vi "App - analyze RUS V6.vi"() -> ()   [LabVIEW 2015] (continued)
CO22__130814c/5_Cooling_2nd_try/September_2014/091614/117.62100K_500_2500_2.10000V_0.00000T_Sep16-2014__20-07-41_001_091614.bin", "last mod"=timestamp(3493757261 s since 1904-01-01), "file name str"="D:\\Data\\Ultrasound\\LSCO\\LSCO22__130814c\\5_Cooling_2nd_try\\September_2014\\091614\\117.62100K_500_2500_2.10000V_0.00000T_Sep16-2014__20-07-41_001_091614.bin", "mod time(min)"=58229287.68333333, "file format"=enum."binary", "power(V)"=2.1, "Magn Field(T) "=0.0}, {"temperature"=117.382, "temperature str"="117.38200", "file path"=path "D:/Data/Ultrasound/LSCO/LSCO22__130814c/5_Cooling_2nd_try/September_2014/091614/117.38200K_500_2500_2.10000V_0.00000T_Sep16-2014__20-09-01_001_091614.bin", "last mod"=timestamp(3493757341 s since 1904-01-01), "file name str"="D:\\Data\\Ultrasound\\LSCO\\LSCO22__130814c\\5_Cooling_2nd_try\\September_2014\\091614\\117.38200K_500_2500_2.10000V_0.00000T_Sep16-2014__20-09-01_001_091614.bin", "mod time(min)"=58229289.016666666, "file format"=enum."binary", "power(V)"=2.1, "Magn Field(T) "=0.0}, {"temperature"=117.138, "temperature str"="117.13800", "file path"=path "D:/Data/Ultrasound/LSCO/LSCO22__130814c/5_Cooling_2nd_try/September_2014/091614/117.13800K_500_2500_2.10000V_0.00000T_Sep16-2014__20-10-20_001_091614.bin", "last mod"=timestamp(3493757420 s since 1904-01-01), "file name str"="D:\\Data\\Ultrasound\\LSCO\\LSCO22__130814c\\5_Cooling_2nd_try\\September_2014\\091614\\117.13800K_500_2500_2.10000V_0.00000T_Sep16-2014__20-10-20_001_091614.bin", "mod time(min)"=58229290.333333336, "file format"=enum."binary", "power(V)"=2.1, "Magn Field(T) "=0.0}, {"temperature"=116.892, "temperature str"="116.89200", "file path"=path "D:/Data/Ultrasound/LSCO/LSCO22__130814c/5_Cooling_2nd_try/September_2014/091614/116.89200K_500_2500_2.10000V_0.00000T_Sep16-2014__20-11-40_001_091614.bin", "last mod"=timestamp(3493757500 s since 1904-01-01), "file name str"="D:\\Data\\Ultrasound\\LSCO\\LSCO22__130814c\\5_Cooling_2nd_try\\September_2014\\091614\\116.89200K_500_2500_2.10000V_0.00000T_Sep16-2014__20-11-40_001_091614.bin", "mod time(min)"=58229291.666666664, "file format"=enum."binary", "power(V)"=2.1, "Magn Field(T) "=0.0}, {"temperature"=116.657, "temperature str"="116.65700", "file path"=path "D:/Data/Ultrasound/LSCO/LSCO22__130814c/5_Cooling_2nd_try/September_2014/091614/116.65700K_500_2500_2.10000V_0.00000T_Sep16-2014__20-12-59_001_091614.bin", "last mod"=timestamp(3493757579 s since 1904-01-01), "file name str"="D:\\Data\\Ultrasound\\LSCO\\LSCO22__130814c\\5_Cooling_2nd_try\\September_2014\\091614\\116.65700K_500_2500_2.10000V_0.00000T_Sep16-2014__20-12-59_001_091614.bin", "mod time(min)"=58229292.983333334, "file format"=enum."binary", "power(V)"=2.1, "Magn Field(T) "=0.0}, {"temperature"=116.414, "temperature str"="116.41400", "file path"=path "D:/Data/Ultrasound/LSCO/LSCO22__130814c/5_Cooling_2nd_try/September_2014/091614/116.41400K_500_2500_2.10000V_0.00000T_Sep16-2014__20-14-18_001_091614.bin", "last mod"=timestamp(3493757658 s since 1904-01-01), "file name str"="D:\\Data\\Ultrasound\\LSCO\\LSCO22__130814c\\5_Cooling_2nd_try\\September_2014\\091614\\116.41400K_500_2500_2.10000V_0.00000T_Sep16-2014__20-14-18_001_091614.bin", "mod time(min)"=58229294.3, "file format"=enum."binary", "power(V)"=2.1, "Magn Field(T) "=0.0}, {"temperature"=116.182, "temperature str"="116.18200", "file path"=path "D:/Data/Ultrasound/LSCO/LSCO22__130814c/5_Cooling_2nd_try/September_2014/091614/116.18200K_500_2500_2.10000V_0.00000T_Sep16-2014__20-15-38_001_091614.bin", "last mod"=timestamp(3493757738 s since 1904-01-01), "file name str"="D:\\Data\\Ultrasound\\LSCO\\LSCO22__130814c\\5_Cooling_2nd_try\\September_2014\\091614\\116.18200K_500_2500_2.10000V_0.00000T_Sep16-2014__20-15-38_001_091614.bin", "mod time(min)"=58229295.63333333, "file format"=enum."binary", "power(V)"=2.1, "Magn Field(T) "=0.0}, {"temperature"=115.94, "temperature str"="115.94000", "file path"=path "D:/Data/Ultrasound/LSCO/LSCO22__130814c/5_Cooling_2nd_try/September_2014/091614/115.94000K_500_2500_2.10000V_0.00000T_Sep16-2014__20-16-57_001_091614.bin", "last mod"=timestamp(3493757817 s since 1904-01-01), "file name str"="D:\\Data\\Ultrasound\\LSCO\\LSCO22__130814c\\5_Cooling_2nd_try\\September_2014\\091614\\115.94000K_500_2500_2.10000V_0.00000T_Sep16-2014__20-16-57_001_091614.bin", "mod time(min)"=58229296.95, "file format"=enum."binary", "power(V)"=2.1, "Magn Field(T) "=0.0}, {"temperature"=115.7, "temperature str"="115.70000", "file path"=path "D:/Data/Ultrasound/LSCO/LSCO22__130814c/5_Cooling_2nd_try/September_2014/091614/115.70000K_500_2500_2.10000V_0.00000T_Sep16-2014__20-18-16_001_091614.bin", "last mod"=timestamp(3493757896 s since 1904-01-01), "file name str"="D:\\Data\\Ultrasound\\LSCO\\LSCO22__130814c\\5_Cooling_2nd_try\\September_2014\\091614\\115.70000K_500_2500_2.10000V_0.00000T_Sep16-2014__20-18-16_001_091614.bin", "mod time(min)"=58229298.266666666, "file format"=enum."binary", "power(V)"=2.1, "Magn Field(T) "=0.0}, {"temperature"=115.472, "temperature str"="115.47200", "file path"=path "D:/Data/Ultrasound/LSCO/LSCO22__130814c/5_Cooling_2nd_try/September_2014/091614/115.47200K_500_2500_2.10000V_0.00000T_Sep16-2014__20-19-36_001_091614.bin", "last mod"=timestamp(3493757976 s since 1904-01-01), "file name str"="D:\\Data\\Ultrasound\\LSCO\\LSCO22__130814c\\5_Cooling_2nd_try\\September_2014\\091614\\115.47200K_500_2500_2.10000V_0.00000T_Sep16-2014__20-19-36_001_091614.bin", "mod time(min)"=58229299.6, "file format"=enum."binary", "power(V)"=2.1, "Magn Field(T) "=0.0}, {"temperature"=115.231, "temperature str"="115.23100", "file path"=path "D:/Data/Ultrasound/LSCO/LSCO22__130814c/5_Cooling_2nd_try/September_2014/091614/115.23100K_500_2500_2.10000V_0.00000T_Sep16-2014__20-20-55_001_091614.bin", "last mod"=timestamp(3493758055 s since 1904-01-01), "file name str"="D:\\Data\\Ultrasound\\LSCO\\LSCO22__130814c\\5_Cooling_2nd_try\\September_2014\\091614\\115.23100K_500_2500_2.10000V_0.00000T_Sep16-2014__20-20-55_001_091614.bin", "mod time(min)"=58229300.916666664, "file format"=enum."binary", "power(V)"=2.1, "Magn Field(T) "=0.0}, {"temperature"=115.003, "temperature str"="115.00300", "file path"=path "D:/Data/Ultrasound/LSCO/LSCO22__130814c/5_Cooling_2nd_try/September_2014/091614/115.00300K_500_2500_2.10000V_0.00000T_Sep16-2014__20-22-15_001_091614.bin", "last mod"=timestamp(3493758135 s since 1904-01-01), "file name str"="D:\\Data\\Ultrasound\\LSCO\\LSCO22__130814c\\5_Cooling_2nd_try\\September_2014\\091614\\115.00300K_500_2500_2.10000V_0.00000T_Sep16-2014__20-22-15_001_091614.bin", "mod time(min)"=58229302.25, "file format"=enum."binary", "power(V)"=2.1, "Magn Field(T) "=0.0}, {"temperature"=114.767, "temperature str"="114.76700", "file path"=path "D:/Data/Ultrasound/LSCO/LSCO22__130814c/5_Cooling_2nd_try/September_2014/091614/114.76700K_500_2500_2.10000V_0.00000T_Sep16-2014__20-23-34_001_091614.bin", "last mod"=timestamp(3493758214 s since 1904-01-01), "file name str"="D:\\Data\\Ultrasound\\LSCO\\LSCO22__130814c\\5_Cooling_2nd_try\\September_2014\\091614\\114.76700K_500_2500_2.10000V_0.00000T_Sep16-2014__20-23-34_001_091614.bin", "mod time(min)"=58229303.56666667, "file format"=enum."binary", "power(V)"=2.1, "Magn Field(T) "=0.0}, {"temperature"=114.531, "temperature str"="114.53100", "file path"=path "D:/Data/Ultrasound/LSCO/LSCO22__130814c/5_Cooling_2nd_try/September_2014/091614/114.53100K_500_2500_2.10000V_0.00000T_Sep16-2014__20-24-53_001_091614.bin", "last mod"=timestamp(3493758293 s since 1904-01-01), "file name str"="D:\\Data\\Ultrasound\\LSCO\\LSCO22__130814c\\5_Cooling_2nd_try\\September_2014\\091614\\114.53100K_500_2500_2.10000V_0.00000T_Sep16-2014__20-24-53_001_091614.bin", "mod time(min)"=58229304.88333333, "file format"=enum."binary", "power(V)"=2.1, "Magn Field(T) "=0.0}, {"temperature"=114.307, "temperature str"="114.30700", "file path"=path "D:/Data/Ultrasound/LSCO/LSCO22__130814c/5_Cooling_2nd_try/September_2014/091614/114.30700K_500_2500_2.10000V_0.00000T_Sep16-2014__20-26-13_001_091614.bin", "last mod"=timestamp(3493758373 s since 1904-01-01), "file name str"="D:\\Data\\Ultrasound\\LSCO\\LSCO22__130814c\\5_Cooling_2nd_try\\September_2014\\091614\\114.30700K_500_2500_2.10000V_0.00000T_Sep16-2014__20-26-13_001_091614.bin", "mod time(min)"=58229306.21666667, "file format"=enum."binary", "power(V)"=2.1, "Magn Field(T) "=0.0}, {"temperature"=114.072, "temperature str"="114.07200", "file path"=path "D:/Data/Ultrasound/LSCO/LSCO22__130814c/5_Cooling_2nd_try/September_2014/091614/114.07200K_500_2500_2.10000V_0.00000T_Sep16-2014__20-27-32_001_091614.bin", "last mod"=timestamp(3493758452 s since 1904-01-01), "file name str"="D:\\Data\\Ultrasound\\LSCO\\LSCO22__130814c\\5_Cooling_2nd_try\\September_2014\\091614\\114.07200K_500_2500_2.10000V_0.00000T_Sep16-2014__20-27-32_001_091614.bin", "mod time(min)"=58229307.53333333, "file format"=enum."binary", "power(V)"=2.1, "Magn Field(T) "=0.0}, {"temperature"=113.842, "temperature str"="113.84200", "file path"=path "D:/Data/Ultrasound/LSCO/LSCO22__130814c/5_Cooling_2nd_try/September_2014/091614/113.84200K_500_2500_2.10000V_0.00000T_Sep16-2014__20-28-52_001_091614.bin", "last mod"=timestamp(3493758532 s since 1904-01-01), "file name str"="D:\\Data\\Ultrasound\\LSCO\\LSCO22__130814c\\5_Cooling_2nd_try\\September_2014\\091614\\113.84200K_500_2500_2.10000V_0.00000T_Sep16-2014__20-28-52_001_091614.bin", "mod time(min)"=58229308.86666667, "file format"=enum."binary", "power(V)"=2.1, "Magn Field(T) "=0.0}, {"temperature"=113.618, "temperature str"="113.61800", "file path"=path "D:/Data/Ultrasound/LSCO/LSCO22__130814c/5_Cooling_2nd_try/September_2014/091614/113.61800K_500_2500_2.10000V_0.00000T_Sep16-2014__20-30-11_001_091614.bin", "last mod"=timestamp(3493758611 s since 1904-01-01), "file name str"="D:\\Data\\Ultrasound\\LSCO\\LSCO22__130814c\\5_Cooling_2nd_try\\September_2014\\091614\\113.61800K_500_2500_2.10000V_0.00000T_Sep16-2014__20-30-11_001_091614.bin", "mod time(min)"=58229310.18333333, "file format"=enum."binary", "power(V)"=2.1, "Magn Field(T) "=0.0}, {"temperature"=113.387, "temperature str"="113.38700", "file path"=path "D:/Data/Ultrasound/LSCO/LSCO22__130814c/5_Cooling_2nd_try/September_2014/091614/113.38700K_500_2500_2.10000V_0.00000T_Sep16-2014__20-31-30_001_091614.bin", "last mod"=timestamp(3493758690 s since 1904-01-01), "file name str"="D:\\Data\\Ultrasound\\LSCO\\LSCO22__130814c\\5_Cooling_2nd_try\\September_2014\\091614\\113.38700K_500_2500_2.10000V_0.00000T_Sep16-2014__20-31-30_001_091614.bin", "mod time(min)"=58229311.5, "file format"=enum."binary", "power(V)"=2.1, "Magn Field(T) "=0.0}, {"temperature"=113.167, "temperature str"="113.16700", "file path"=path "D:/Data/Ultrasound/LSCO/LSCO22__130814c/5_Cooling_2nd_try/September_2014/091614/113.16700K_500_2500_2.10000V_0.00000T_Sep16-2014__20-32-49_001_091614.bin", "last mod"=timestamp(3493758769 s since 1904-01-01), "file name str"="D:\\Data\\Ultrasound\\LSCO\\LSCO22__130814c\\5_Cooling_2nd_try\\September_2014\\091614\\113.16700K_500_2500_2.10000V_0.00000T_Sep16-2014__20-32-49_001_091614.bin", "mod time(min)"=58229312.81666667, "file format"=enum."binary", "power(V)"=2.1, "Magn Field(T) "=0.0}, {"temperature"=112.937, "temperature str"="112.93700", "file path"=path "D:/Data/Ultrasound/LSCO/LSCO22__130814c/5_Cooling_2nd_try/September_2014/091614/112.93700K_500_2500_2.10000V_0.00000T_Sep16-2014__20-34-09_001_091614.bin", "last mod"=timestamp(3493758849 s since 1904-01-01), "file name str"="D:\\Data\\Ultrasound\\LSCO\\LSCO22__130814c\\5_Cooling_2nd_try\\September_2014\\091614\\112.93700K_500_2500_2.10000V_0.00000T_Sep16-2014__20-34-09_001_091614.bin", "mod time(min)"=58229314.15, "file format"=enum."binary", "power(V)"=2.1, "Magn Field(T) "=0.0}, {"temperature"=112.71, "temperature str"="112.71000", "file path"=path "D:/Data/Ultrasound/LSCO/LSCO22__130814c/5_Cooling_2nd_try/September_2014/091614/112.71000K_500_2500_2.10000V_0.00000T_Sep16-2014__20-35-28_001_091614.bin", "last mod"=timestamp(3493758928 s since 1904-01-01), "file name str"="D:\\Data\\Ultrasound\\LSCO\\LSCO22__130814c\\5_Cooling_2nd_try\\September_2014\\091614\\112.71000K_500_2500_2.10000V_0.00000T_Sep16-2014__20-35-28_001_091614.bin", "mod time(min)"=58229315.46666667, "file format"=enum."binary", "power(V)"=2.1, "Magn Field(T) "=0.0}, {"temperature"=112.492, "temperature str"="112.49200", "file path"=path "D:/Data/Ultrasound/LSCO/LSCO22__130814c/5_Cooling_2nd_try/September_2014/091614/112.49200K_500_2500_2.10000V_0.00000T_Sep16-2014__20-36-47_001_091614.bin", "last mod"=timestamp(3493759007 s since 1904-01-01), "file name str"="D:\\Data\\Ultrasound\\LSCO\\LSCO22__130814c\\5_Cooling_2nd_try\\September_2014\\091614\\112.49200K_500_2500_2.10000V_0.00000T_Sep16-2014__20-36-47_001_091614.bin", "mod time(min)"=58229316.78333333, "file format"=enum."binary", "power(V)"=2.1, "Magn Field(T) "=0.0}, {"temperature"=112.266, "temperature str"="112.26600", "file path"=path "D:/Data/Ultrasound/LSCO/LSCO22__130814c/5_Cooling_2nd_try/September_2014/091614/112.26600K_500_2500_2.10000V_0.00000T_Sep16-2014__20-38-07_001_091614.bin", "last mod"=timestamp(3493759087 s since 1904-01-01), "file name str"="D:\\Data\\Ultrasound\\LSCO\\LSCO22__130814c\\5_Cooling_2nd_try\\September_2014\\091614\\112.26600K_500_2500_2.10000V_0.00000T_Sep16-2014__20-38-07_001_091614.bin", "mod time(min)"=58229318.11666667, "file format"=enum."binary", "power(V)"=2.1, "Magn Field(T) "=0.0}, {"temperature"=112.049, "temperature str"="112.04900", "file path"=path "D:/Data/Ultrasound/LSCO/LSCO22__130814c/5_Cooling_2nd_try/September_2014/091614/112.04900K_500_2500_2.10000V_0.00000T_Sep16-2014__20-39-26_001_091614.bin", "last mod"=timestamp(3493759166 s since 1904-01-01), "file name str"="D:\\Data\\Ultrasound\\LSCO\\LSCO22__130814c\\5_Cooling_2nd_try\\September_2014\\091614\\112.04900K_500_2500_2.10000V_0.00000T_Sep16-2014__20-39-26_001_091614.bin", "mod time(min)"=58229319.43333333, "file format"=enum."binary", "power(V)"=2.1, "Magn Field(T) "=0.0}, {"temperature"=111.826, "temperature str"="111.82600", "file path"=path "D:/Data/Ultrasound/LSCO/LSCO22__130814c/5_Cooling_2nd_try/September_2014/091614/111.82600K_500_2500_2.10000V_0.00000T_Sep16-2014__20-40-45_001_091614.bin", "last mod"=timestamp(3493759245 s since 1904-01-01), "file name str"="D:\\Data\\Ultrasound\\LSCO\\LSCO22__130814c\\5_Cooling_2nd_try\\September_2014\\091614\\111.82600K_500_2500_2.10000V_0.00000T_Sep16-2014__20-40-45_001_091614.bin", "mod time(min)"=58229320.75, "file format"=enum."binary", "power(V)"=2.1, "Magn Field(T) "=0.0}, {"temperature"=111.603, "temperature str"="111.60300", "file path"=path "D:/Data/Ultrasound/LSCO/LSCO22__130814c/5_Cooling_2nd_try/September_2014/091614/111.60300K_500_2500_2.10000V_0.00000T_Sep16-2014__20-42-05_001_091614.bin", "last mod"=timestamp(3493759325 s since 1904-01-01), "file name str"="D:\\Data\\Ultrasound\\LSCO\\LSCO22__130814c\\5_Cooling_2nd_try\\September_2014\\091614\\111.60300K_500_2500_2.10000V_0.00000T_Sep16-2014__20-42-05_001_091614.bin", "mod time(min)"=58229322.083333336, "file format"=enum."binary", "power(V)"=2.1, "Magn Field(T) "=0.0}, {"temperature"=111.388, "temperature str"="111.38800", "file path"=path "D:/Data/Ultrasound/LSCO/LSCO22__130814c/5_Cooling_2nd_try/September_2014/091614/111.38800K_500_2500_2.10000V_0.00000T_Sep16-2014__20-43-24_001_091614.bin", "last mod"=timestamp(3493759404 s since 1904-01-01), "file name str"="D:\\Data\\Ultrasound\\LSCO\\LSCO22__130814c\\5_Cooling_2nd_try\\September_2014\\091614\\111.38800K_500_2500_2.10000V_0.00000T_Sep16-2014__20-43-24_001_091614.bin", "mod time(min)"=58229323.4, "file format"=enum."binary", "power(V)"=2.1, "Magn Field(T) "=0.0}, {"temperature"=111.168, "temperature str"="111.16800", "file path"=path "D:/Data/Ultrasound/LSCO/LSCO22__130814c/5_Cooling_2nd_try/September_2014/091614/111.16800K_500_2500_2.10000V_0.00000T_Sep16-2014__20-44-44_001_091614.bin", "last mod"=timestamp(3493759484 s since 1904-01-01), "file name str"="D:\\Data\\Ultrasound\\LSCO\\LSCO22__130814c\\5_Cooling_2nd_try\\September_2014\\091614\\111.16800K_500_2500_2.10000V_0.00000T_Sep16-2014__20-44-44_001_091614.bin", "mod time(min)"=58229324.733333334, "file format"=enum."binary", "power(V)"=2.1, "Magn Field(T) "=0.0}, {"temperature"=110.956, "temperature str"="110.95600", "file path"=path "D:/Data/Ultrasound/LSCO/LSCO22__130814c/5_Cooling_2nd_try/September_2014/091614/110.95600K_500_2500_2.10000V_0.00000T_Sep16-2014__20-46-03_001_091614.bin", "last mod"=timestamp(3493759563 s since 1904-01-01), "file name str"="D:\\Data\\Ultrasound\\LSCO\\LSCO22__130814c\\5_Cooling_2nd_try\\September_2014\\091614\\110.95600K_500_2500_2.10000V_0.00000T_Sep16-2014__20-46-03_001_091614.bin", "mod time(min)"=58229326.05, "file format"=enum."binary", "power(V)"=2.1, "Magn Field(T) "=0.0}, {"temperature"=110.737, "temperature str"="110.73700", "file path"=path "D:/Data/Ultrasound/LSCO/LSCO22__130814c/5_Cooling_2nd_try/September_2014/091614/110.73700K_500_2500_2.10000V_0.00000T_Sep16-2014__20-47-22_001_091614.bin", "last mod"=timestamp(3493759642 s since 1904-01-01), "file name str"="D:\\Data\\Ultrasound\\LSCO\\LSCO22__130814c\\5_Cooling_2nd_try\\September_2014\\091614\\110.73700K_500_2500_2.10000V_0.00000T_Sep16-2014__20-47-22_001_091614.bin", "mod time(min)"=58229327.36666667, "file format"=enum."binary", "power(V)"=2.1, "Magn Field(T) "=0.0}, {"temperature"=110.519, "temperature str"="110.51900", "file path"=path "D:/Data/Ultrasound/LSCO/LSCO22__130814c/5_Cooling_2nd_try/September_2014/091614/110.51900K_500_2500_2.10000V_0.00000T_Sep16-2014__20-48-42_001_091614.bin", "last mod"=timestamp(3493759722 s since 1904-01-01), "file name str"="D:\\Data\\Ultrasound\\LSCO\\LSCO22__130814c\\5_Cooling_2nd_try\\September_2014\\091614\\110.51900K_500_2500_2.10000V_0.00000T_Sep16-2014__20-48-42_001_091614.bin", "mod time(min)"=58229328.7, "file format"=enum."binary", "power(V)"=2.1, "Magn Field(T) "=0.0}, {"temperature"=110.309, "temperature str"="110.30900", "file path"=path "D:/Data/Ultrasound/LSCO/LSCO22__130814c/5_Cooling_2nd_try/September_2014/091614/110.30900K_500_2500_2.10000V_0.00000T_Sep16-2014__20-50-01_001_091614.bin", "last mod"=timestamp(3493759801 s since 1904-01-01), "file name str"="D:\\Data\\Ultrasound\\LSCO\\LSCO22__130814c\\5_Cooling_2nd_try\\September_2014\\091614\\110.30900K_500_2500_2.10000V_0.00000T_Sep16-2014__20-50-01_001_091614.bin", "mod time(min)"=58229330.016666666, "file format"=enum."binary", "power(V)"=2.1, "Magn Field(T) "=0.0}, {"temperature"=110.092, "temperature str"="110.09200", "file path"=path "D:/Data/Ultrasound/LSCO/LSCO22__130814c/5_Cooling_2nd_try/September_2014/091614/110.09200K_500_2500_2.10000V_0.00000T_Sep16-2014__20-51-20_001_091614.bin", "last mod"=timestamp(3493759880 s since 1904-01-01), "file name str"="D:\\Data\\Ultrasound\\LSCO\\LSCO22__130814c\\5_Cooling_2nd_try\\September_2014\\091614\\110.09200K_500_2500_2.10000V_0.00000T_Sep16-2014__20-51-20_001_091614.bin", "mod time(min)"=58229331.333333336, "file format"=enum."binary", "power(V)"=2.1, "Magn Field(T) "=0.0}, {"temperature"=109.886, "temperature str"="109.88600", "file path"=path "D:/Data/Ultrasound/LSCO/LSCO22__130814c/5_Cooling_2nd_try/September_2014/091614/109.88600K_500_2500_2.10000V_0.00000T_Sep16-2014__20-52-40_001_091614.bin", "last mod"=timestamp(3493759960 s since 1904-01-01), "file name str"="D:\\Data\\Ultrasound\\LSCO\\LSCO22__130814c\\5_Cooling_2nd_try\\September_2014\\091614\\109.88600K_500_2500_2.10000V_0.00000T_Sep16-2014__20-52-40_001_091614.bin", "mod time(min)"=58229332.666666664, "file format"=enum."binary", "power(V)"=2.1, "Magn Field(T) "=0.0}, {"temperature"=109.672, "temperature str"="109.67200", "file path"=path "D:/Data/Ultrasound/LSCO/LSCO22__130814c/5_Cooling_2nd_try/September_2014/091614/109.67200K_500_2500_2.10000V_0.00000T_Sep16-2014__20-53-59_001_091614.bin", "last mod"=timestamp(3493760039 s since 1904-01-01), "file name str"="D:\\Data\\Ultrasound\\LSCO\\LSCO22__130814c\\5_Cooling_2nd_try\\September_2014\\091614\\109.67200K_500_2500_2.10000V_0.00000T_Sep16-2014__20-53-59_001_091614.bin", "mod time(min)"=58229333.983333334, "file format"=enum."binary", "power(V)"=2.1, "Magn Field(T) "=0.0}, {"temperature"=109.459, "temperature str"="109.45900", "file path"=path "D:/Data/Ultrasound/LSCO/LSCO22__130814c/5_Cooling_2nd_try/September_2014/091614/109.45900K_500_2500_2.10000V_0.00000T_Sep16-2014__20-55-19_001_091614.bin", "last mod"=timestamp(3493760119 s since 1904-01-01), "file name str"="D:\\Data\\Ultrasound\\LSCO\\LSCO22__130814c\\5_Cooling_2nd_try\\September_2014\\091614\\109.45900K_500_2500_2.10000V_0.00000T_Sep16-2014__20-55-19_001_091614.bin", "mod time(min)"=58229335.31666667, "file format"=enum."binary", "power(V)"=2.1, "Magn Field(T) "=0.0}, {"temperature"=109.253, "temperature str"="109.25300", "file path"=path "D:/Data/Ultrasound/LSCO/LSCO22__130814c/5_Cooling_2nd_try/September_2014/091614/109.25300K_500_2500_2.10000V_0.00000T_Sep16-2014__20-56-38_001_091614.bin", "last mod"=timestamp(3493760198 s since 1904-01-01), "file name str"="D:\\Data\\Ultrasound\\LSCO\\LSCO22__130814c\\5_Cooling_2nd_try\\September_2014\\091614\\109.25300K_500_2500_2.10000V_0.00000T_Sep16-2014__20-56-38_001_091614.bin", "mod time(min)"=58229336.63333333, "file format"=enum."binary", "power(V)"=2.1, "Magn Field(T) "=0.0}, {"temperature"=109.04, "temperature str"="109.04000", "file path"=path "D:/Data/Ultrasound/LSCO/LSCO22__130814c/5_Cooling_2nd_try/September_2014/091614/109.04000K_500_2500_2.10000V_0.00000T_Sep16-2014__20-57-57_001_091614.bin", "last mod"=timestamp(3493760277 s since 1904-01-01), "file name str"="D:\\Data\\Ultrasound\\LSCO\\LSCO22__130814c\\5_Cooling_2nd_try\\September_2014\\091614\\109.04000K_500_2500_2.10000V_0.00000T_Sep16-2014__20-57-57_001_091614.bin", "mod time(min)"=58229337.95, "file format"=enum."binary", "power(V)"=2.1, "Magn Field(T) "=0.0}, {"temperature"=108.839, "temperature str"="108.83900", "file path"=path "D:/Data/Ultrasound/LSCO/LSCO22__130814c/5_Cooling_2nd_try/September_2014/091614/108.83900K_500_2500_2.10000V_0.00000T_Sep16-2014__20-59-17_001_091614.bin", "last mod"=timestamp(3493760357 s since 1904-01-01), "file name str"="D:\\Data\\Ultrasound\\LSCO\\LSCO22__130814c\\5_Cooling_2nd_try\\September_2014\\091614\\108.83900K_500_2500_2.10000V_0.00000T_Sep16-2014__20-59-17_001_091614.bin", "mod time(min)"=58229339.28333333, "file format"=enum."binary", "power(V)"=2.1, "Magn Field(T) "=0.0}, {"temperature"=108.626, "temperature str"="108.62600", "file path"=path "D:/Data/Ultrasound/LSCO/LSCO22__130814c/5_Cooling_2nd_try/September_2014/091614/108.62600K_500_2500_2.10000V_0.00000T_Sep16-2014__21-00-36_001_091614.bin", "last mod"=timestamp(3493760436 s since 1904-01-01), "file name str"="D:\\Data\\Ultrasound\\LSCO\\LSCO22__130814c\\5_Cooling_2nd_try\\September_2014\\091614\\108.62600K_500_2500_2.10000V_0.00000T_Sep16-2014__21-00-36_001_091614.bin", "mod time(min)"=58229340.6, "file format"=enum."binary", "power(V)"=2.1, "Magn Field(T) "=0.0}, {"temperature"=108.42, "temperature str"="108.42000", "file path"=path "D:/Data/Ultrasound/LSCO/LSCO22__130814c/5_Cooling_2nd_try/September_2014/091614/108.42000K_500_2500_2.10000V_0.00000T_Sep16-2014__21-01-55_001_091614.bin", "last mod"=timestamp(3493760515 s since 1904-01-01), "file name str"="D:\\Data\\Ultrasound\\LSCO\\LSCO22__130814c\\5_Cooling_2nd_try\\September_2014\\091614\\108.42000K_500_2500_2.10000V_0.00000T_Sep16-2014__21-01-55_001_091614.bin", "mod time(min)"=58229341.916666664, "file format"=enum."binary", "power(V)"=2.1, "Magn Field(T) "=0.0}, {"temperature"=108.218, "temperature str"="108.21800", "file path"=path "D:/Data/Ultrasound/LSCO/LSCO22__130814c/5_Cooling_2nd_try/September_2014/091614/108.21800K_500_2500_2.10000V_0.00000T_Sep16-2014__21-03-15_001_091614.bin", "last mod"=timestamp(3493760595 s since 1904-01-01), "file name str"="D:\\Data\\Ultrasound\\LSCO\\LSCO22__130814c\\5_Cooling_2nd_try\\September_2014\\091614\\108.21800K_500_2500_2.10000V_0.00000T_Sep16-2014__21-03-15_001_091614.bin", "mod time(min)"=58229343.25, "file format"=enum."binary", "power(V)"=2.1, "Magn Field(T) "=0.0}, {"temperature"=108.011, "temperature str"="108.01100", "file path"=path "D:/Data/Ultrasound/LSCO/LSCO22__130814c/5_Cooling_2nd_try/September_2014/091614/108.01100K_500_2500_2.10000V_0.00000T_Sep16-2014__21-04-34_001_091614.bin", "last mod"=timestamp(3493760674 s since 1904-01-01), "file name str"="D:\\Data\\Ultrasound\\LSCO\\LSCO22__130814c\\5_Cooling_2nd_try\\September_2014\\091614\\108.01100K_500_2500_2.10000V_0.00000T_Sep16-2014__21-04-34_001_091614.bin", "mod time(min)"=58229344.56666667, "file format"=enum."binary", "power(V)"=2.1, "Magn Field(T) "=0.0}, {"temperature"=107.814, "temperature str"="107.81400", "file path"=path "D:/Data/Ultrasound/LSCO/LSCO22__130814c/5_Cooling_2nd_try/September_2014/091614/107.81400K_500_2500_2.10000V_0.00000T_Sep16-2014__21-05-54_001_091614.bin", "last mod"=timestamp(3493760754 s since 1904-01-01), "file name str"="D:\\Data\\Ultrasound\\LSCO\\LSCO22__130814c\\5_Cooling_2nd_try\\September_2014\\091614\\107.81400K_500_2500_2.10000V_0.00000T_Sep16-2014__21-05-54_001_091614.bin", "mod time(min)"=58229345.9, "file format"=enum."binary", "power(V)"=2.1, "Magn Field(T) "=0.0}, {"temperature"=107.607, "temperature str"="107.60700", "file path"=path "D:/Data/Ultrasound/LSCO/LSCO22__130814c/5_Cooling_2nd_try/September_2014/091614/107.60700K_500_2500_2.10000V_0.00000T_Sep16-2014__21-07-13_001_091614.bin", "last mod"=timestamp(3493760833 s since 1904-01-01), "file name str"="D:\\Data\\Ultrasound\\LSCO\\LSCO22__130814c\\5_Cooling_2nd_try\\September_2014\\091614\\107.60700K_500_2500_2.10000V_0.00000T_Sep16-2014__21-07-13_001_091614.bin", "mod time(min)"=58229347.21666667, "file format"=enum."binary", "power(V)"=2.1, "Magn Field(T) "=0.0}, {"temperature"=107.403, "temperature str"="107.40300", "file path"=path "D:/Data/Ultrasound/LSCO/LSCO22__130814c/5_Cooling_2nd_try/September_2014/091614/107.40300K_500_2500_2.10000V_0.00000T_Sep16-2014__21-08-32_001_091614.bin", "last mod"=timestamp(3493760912 s since 1904-01-01), "file name str"="D:\\Data\\Ultrasound\\LSCO\\LSCO22__130814c\\5_Cooling_2nd_try\\September_2014\\091614\\107.40300K_500_2500_2.10000V_0.00000T_Sep16-2014__21-08-32_001_091614.bin", "mod time(min)"=58229348.53333333, "file format"=enum."binary", "power(V)"=2.1, "Magn Field(T) "=0.0}, {"temperature"=107.207, "temperature str"="107.20700", "file path"=path "D:/Data/Ultrasound/LSCO/LSCO22__130814c/5_Cooling_2nd_try/September_2014/091614/107.20700K_500_2500_2.10000V_0.00000T_Sep16-2014__21-09-52_001_091614.bin", "last mod"=timestamp(3493760992 s since 1904-01-01), "file name str"="D:\\Data\\Ultrasound\\LSCO\\LSCO22__130814c\\5_Cooling_2nd_try\\September_2014\\091614\\107.20700K_500_2500_2.10000V_0.00000T_Sep16-2014__21-09-52_001_091614.bin", "mod time(min)"=58229349.86666667, "file format"=enum."binary", "power(V)"=2.1, "Magn Field(T) "=0.0}, {"temperature"=107.004, "temperature str"="107.00400", "file path"=path "D:/Data/Ultrasound/LSCO/LSCO22__130814c/5_Cooling_2nd_try/September_2014/091614/107.00400K_500_2500_2.10000V_0.00000T_Sep16-2014__21-11-11_001_091614.bin", "last mod"=timestamp(3493761071 s since 1904-01-01), "file name str"="D:\\Data\\Ultrasound\\LSCO\\LSCO22__130814c\\5_Cooling_2nd_try\\September_2014\\091614\\107.00400K_500_2500_2.10000V_0.00000T_Sep16-2014__21-11-11_001_091614.bin", "mod time(min)"=58229351.18333333, "file format"=enum."binary", "power(V)"=2.1, "Magn Field(T) "=0.0}, {"temperature"=106.803, "temperature str"="106.80300", "file path"=path "D:/Data/Ultrasound/LSCO/LSCO22__130814c/5_Cooling_2nd_try/September_2014/091614/106.80300K_500_2500_2.10000V_0.00000T_Sep16-2014__21-12-30_001_091614.bin", "last mod"=timestamp(3493761150 s since 1904-01-01), "file name str"="D:\\Data\\Ultrasound\\LSCO\\LSCO22__130814c\\5_Cooling_2nd_try\\September_2014\\091614\\106.80300K_500_2500_2.10000V_0.00000T_Sep16-2014__21-12-30_001_091614.bin", "mod time(min)"=58229352.5, "file format"=enum."binary", "power(V)"=2.1, "Magn Field(T) "=0.0}, {"temperature"=106.609, "temperature str"="106.60900", "file path"=path "D:/Data/Ultrasound/LSCO/LSCO22__130814c/5_Cooling_2nd_try/September_2014/091614/106.60900K_500_2500_2.10000V_0.00000T_Sep16-2014__21-13-50_001_091614.bin", "last mod"=timestamp(3493761230 s since 1904-01-01), "file name str"="D:\\Data\\Ultrasound\\LSCO\\LSCO22__130814c\\5_Cooling_2nd_try\\September_2014\\091614\\106.60900K_500_2500_2.10000V_0.00000T_Sep16-2014__21-13-50_001_091614.bin", "mod time(min)"=58229353.833333336, "file format"=enum."binary", "power(V)"=2.1, "Magn Field(T) "=0.0}, {"temperature"=106.409, "temperature str"="106.40900", "file path"=path "D:/Data/Ultrasound/LSCO/LSCO22__130814c/5_Cooling_2nd_try/September_2014/091614/106.40900K_500_2500_2.10000V_0.00000T_Sep16-2014__21-15-09_001_091614.bin", "last mod"=timestamp(3493761309 s since 1904-01-01), "file name str"="D:\\Data\\Ultrasound\\LSCO\\LSCO22__130814c\\5_Cooling_2nd_try\\September_2014\\091614\\106.40900K_500_2500_2.10000V_0.00000T_Sep16-2014__21-15-09_001_091614.bin", "mod time(min)"=58229355.15, "file format"=enum."binary", "power(V)"=2.1, "Magn Field(T) "=0.0}, {"temperature"=106.218, "temperature str"="106.21800", "file path"=path "D:/Data/Ultrasound/LSCO/LSCO22__130814c/5_Cooling_2nd_try/September_2014/091614/106.21800K_500_2500_2.10000V_0.00000T_Sep16-2014__21-16-29_001_091614.bin", "last mod"=timestamp(3493761389 s since 1904-01-01), "file name str"="D:\\Data\\Ultrasound\\LSCO\\LSCO22__130814c\\5_Cooling_2nd_try\\September_2014\\091614\\106.21800K_500_2500_2.10000V_0.00000T_Sep16-2014__21-16-29_001_091614.bin", "mod time(min)"=58229356.483333334, "file format"=enum."binary", "power(V)"=2.1, "Magn Field(T) "=0.0}, {"temperature"=106.019, "temperature str"="106.01900", "file path"=path "D:/Data/Ultrasound/LSCO/LSCO22__130814c/5_Cooling_2nd_try/September_2014/091614/106.01900K_500_2500_2.10000V_0.00000T_Sep16-2014__21-17-48_001_091614.bin", "last mod"=timestamp(3493761468 s since 1904-01-01), "file name str"="D:\\Data\\Ultrasound\\LSCO\\LSCO22__130814c\\5_Cooling_2nd_try\\September_2014\\091614\\106.01900K_500_2500_2.10000V_0.00000T_Sep16-2014__21-17-48_001_091614.bin", "mod time(min)"=58229357.8, "file format"=enum."binary", "power(V)"=2.1, "Magn Field(T) "=0.0}, {"temperature"=105.822, "temperature str"="105.82200", "file path"=path "D:/Data/Ultrasound/LSCO/LSCO22__130814c/5_Cooling_2nd_try/September_2014/091614/105.82200K_500_2500_2.10000V_0.00000T_Sep16-2014__21-19-07_001_091614.bin", "last mod"=timestamp(3493761547 s since 1904-01-01), "file name str"="D:\\Data\\Ultrasound\\LSCO\\LSCO22__130814c\\5_Cooling_2nd_try\\September_2014\\091614\\105.82200K_500_2500_2.10000V_0.00000T_Sep16-2014__21-19-07_001_091614.bin", "mod time(min)"=58229359.11666667, "file format"=enum."binary", "power(V)"=2.1, "Magn Field(T) "=0.0}, {"temperature"=105.631, "temperature str"="105.63100", "file path"=path "D:/Data/Ultrasound/LSCO/LSCO22__130814c/5_Cooling_2nd_try/September_2014/091614/105.63100K_500_2500_2.10000V_0.00000T_Sep16-2014__21-20-27_001_091614.bin", "last mod"=timestamp(3493761627 s since 1904-01-01), "file name str"="D:\\Data\\Ultrasound\\LSCO\\LSCO22__130814c\\5_Cooling_2nd_try\\September_2014\\091614\\105.63100K_500_2500_2.10000V_0.00000T_Sep16-2014__21-20-27_001_091614.bin", "mod time(min)"=58229360.45, "file format"=enum."binary", "power(V)"=2.1, "Magn Field(T) "=0.0}, {"temperature"=105.436, "temperature str"="105.43600", "file path"=path "D:/Data/Ultrasound/LSCO/LSCO22__130814c/5_Cooling_2nd_try/September_2014/091614/105.43600K_500_2500_2.10000V_0.00000T_Sep16-2014__21-21-46_001_091614.bin", "last mod"=timestamp(3493761706 s since 1904-01-01), "file name str"="D:\\Data\\Ultrasound\\LSCO\\LSCO22__130814c\\5_Cooling_2nd_try\\September_2014\\091614\\105.43600K_500_2500_2.10000V_0.00000T_Sep16-2014__21-21-46_001_091614.bin", "mod time(min)"=58229361.766666666, "file format"=enum."binary", "power(V)"=2.1, "Magn Field(T) "=0.0}, {"temperature"=105.248, "temperature str"="105.24800", "file path"=path "D:/Data/Ultrasound/LSCO/LSCO22__130814c/5_Cooling_2nd_try/September_2014/091614/105.24800K_500_2500_2.10000V_0.00000T_Sep16-2014__21-23-05_001_091614.bin", "last mod"=timestamp(3493761785 s since 1904-01-01), "file name str"="D:\\Data\\Ultrasound\\LSCO\\LSCO22__130814c\\5_Cooling_2nd_try\\September_2014\\091614\\105.24800K_500_2500_2.10000V_0.00000T_Sep16-2014__21-23-05_001_091614.bin", "mod time(min)"=58229363.083333336, "file format"=enum."binary", "power(V)"=2.1, "Magn Field(T) "=0.0}, {"temperature"=105.052, "temperature str"="105.05200", "file path"=path "D:/Data/Ultrasound/LSCO/LSCO22__130814c/5_Cooling_2nd_try/September_2014/091614/105.05200K_500_2500_2.10000V_0.00000T_Sep16-2014__21-24-25_001_091614.bin", "last mod"=timestamp(3493761865 s since 1904-01-01), "file name str"="D:\\Data\\Ultrasound\\LSCO\\LSCO22__130814c\\5_Cooling_2nd_try\\September_2014\\091614\\105.05200K_500_2500_2.10000V_0.00000T_Sep16-2014__21-24-25_001_091614.bin", "mod time(min)"=58229364.416666664, "file format"=enum."binary", "power(V)"=2.1, "Magn Field(T) "=0.0}, {"temperature"=104.861, "temperature str"="104.86100", "file path"=path "D:/Data/Ultrasound/LSCO/LSCO22__130814c/5_Cooling_2nd_try/September_2014/091614/104.86100K_500_2500_2.10000V_0.00000T_Sep16-2014__21-25-44_001_091614.bin", "last mod"=timestamp(3493761944 s since 1904-01-01), "file name str"="D:\\Data\\Ultrasound\\LSCO\\LSCO22__130814c\\5_Cooling_2nd_try\\September_2014\\091614\\104.86100K_500_2500_2.10000V_0.00000T_Sep16-2014__21-25-44_001_091614.bin", "mod time(min)"=58229365.733333334, "file format"=enum."binary", "power(V)"=2.1, "Magn Field(T) "=0.0}, {"temperature"=104.676, "temperature str"="104.67600", "file path"=path "D:/Data/Ultrasound/LSCO/LSCO22__130814c/5_Cooling_2nd_try/September_2014/091614/104.67600K_500_2500_2.10000V_0.00000T_Sep16-2014__21-27-04_001_091614.bin", "last mod"=timestamp(3493762024 s since 1904-01-01), "file name str"="D:\\Data\\Ultrasound\\LSCO\\LSCO22__130814c\\5_Cooling_2nd_try\\September_2014\\091614\\104.67600K_500_2500_2.10000V_0.00000T_Sep16-2014__21-27-04_001_091614.bin", "mod time(min)"=58229367.06666667, "file format"=enum."binary", "power(V)"=2.1, "Magn Field(T) "=0.0}, {"temperature"=104.483, "temperature str"="104.48300", "file path"=path "D:/Data/Ultrasound/LSCO/LSCO22__130814c/5_Cooling_2nd_try/September_2014/091614/104.48300K_500_2500_2.10000V_0.00000T_Sep16-2014__21-28-23_001_091614.bin", "last mod"=timestamp(3493762103 s since 1904-01-01), "file name str"="D:\\Data\\Ultrasound\\LSCO\\LSCO22__130814c\\5_Cooling_2nd_try\\September_2014\\091614\\104.48300K_500_2500_2.10000V_0.00000T_Sep16-2014__21-28-23_001_091614.bin", "mod time(min)"=58229368.38333333, "file format"=enum."binary", "power(V)"=2.1, "Magn Field(T) "=0.0}, {"temperature"=104.301, "temperature str"="104.30100", "file path"=path "D:/Data/Ultrasound/LSCO/LSCO22__130814c/5_Cooling_2nd_try/September_2014/091614/104.30100K_500_2500_2.10000V_0.00000T_Sep16-2014__21-29-42_001_091614.bin", "last mod"=timestamp(3493762182 s since 1904-01-01), "file name str"="D:\\Data\\Ultrasound\\LSCO\\LSCO22__130814c\\5_Cooling_2nd_try\\September_2014\\091614\\104.30100K_500_2500_2.10000V_0.00000T_Sep16-2014__21-29-42_001_091614.bin", "mod time(min)"=58229369.7, "file format"=enum."binary", "power(V)"=2.1, "Magn Field(T) "=0.0}, {"temperature"=104.111, "temperature str"="104.11100", "file path"=path "D:/Data/Ultrasound/LSCO/LSCO22__130814c/5_Cooling_2nd_try/September_2014/091614/104.11100K_500_2500_2.10000V_0.00000T_Sep16-2014__21-31-02_001_091614.bin", "last mod"=timestamp(3493762262 s since 1904-01-01), "file name str"="D:\\Data\\Ultrasound\\LSCO\\LSCO22__130814c\\5_Cooling_2nd_try\\September_2014\\091614\\104.11100K_500_2500_2.10000V_0.00000T_Sep16-2014__21-31-02_001_091614.bin", "mod time(min)"=58229371.03333333, "file format"=enum."binary", "power(V)"=2.1, "Magn Field(T) "=0.0}, {"temperature"=103.923, "temperature str"="103.92300", "file path"=path "D:/Data/Ultrasound/LSCO/LSCO22__130814c/5_Cooling_2nd_try/September_2014/091614/103.92300K_500_2500_2.10000V_0.00000T_Sep16-2014__21-32-21_001_091614.bin", "last mod"=timestamp(3493762341 s since 1904-01-01), "file name str"="D:\\Data\\Ultrasound\\LSCO\\LSCO22__130814c\\5_Cooling_2nd_try\\September_2014\\091614\\103.92300K_500_2500_2.10000V_0.00000T_Sep16-2014__21-32-21_001_091614.bin", "mod time(min)"=58229372.35, "file format"=enum."binary", "power(V)"=2.1, "Magn Field(T) "=0.0}, {"temperature"=103.741, "temperature str"="103.74100", "file path"=path "D:/Data/Ultrasound/LSCO/LSCO22__130814c/5_Cooling_2nd_try/September_2014/091614/103.74100K_500_2500_2.10000V_0.00000T_Sep16-2014__21-33-40_001_091614.bin", "last mod"=timestamp(3493762420 s since 1904-01-01), "file name str"="D:\\Data\\Ultrasound\\LSCO\\LSCO22__130814c\\5_Cooling_2nd_try\\September_2014\\091614\\103.74100K_500_2500_2.10000V_0.00000T_Sep16-2014__21-33-40_001_091614.bin", "mod time(min)"=58229373.666666664, "file format"=enum."binary", "power(V)"=2.1, "Magn Field(T) "=0.0}, {"temperature"=103.554, "temperature str"="103.55400", "file path"=path "D:/Data/Ultrasound/LSCO/LSCO22__130814c/5_Cooling_2nd_try/September_2014/091614/103.55400K_500_2500_2.10000V_0.00000T_Sep16-2014__21-35-00_001_091614.bin", "last mod"=timestamp(3493762500 s since 1904-01-01), "file name str"="D:\\Data\\Ultrasound\\LSCO\\LSCO22__130814c\\5_Cooling_2nd_try\\September_2014\\091614\\103.55400K_500_2500_2.10000V_0.00000T_Sep16-2014__21-35-00_001_091614.bin", "mod time(min)"=58229375.0, "file format"=enum."binary", "power(V)"=2.1, "Magn Field(T) "=0.0}, {"temperature"=103.375, "temperature str"="103.37500", "file path"=path "D:/Data/Ultrasound/LSCO/LSCO22__130814c/5_Cooling_2nd_try/September_2014/091614/103.37500K_500_2500_2.10000V_0.00000T_Sep16-2014__21-36-19_001_091614.bin", "last mod"=timestamp(3493762579 s since 1904-01-01), "file name str"="D:\\Data\\Ultrasound\\LSCO\\LSCO22__130814c\\5_Cooling_2nd_try\\September_2014\\091614\\103.37500K_500_2500_2.10000V_0.00000T_Sep16-2014__21-36-19_001_091614.bin", "mod time(min)"=58229376.31666667, "file format"=enum."binary", "power(V)"=2.1, "Magn Field(T) "=0.0}, {"temperature"=103.189, "temperature str"="103.18900", "file path"=path "D:/Data/Ultrasound/LSCO/LSCO22__130814c/5_Cooling_2nd_try/September_2014/091614/103.18900K_500_2500_2.10000V_0.00000T_Sep16-2014__21-37-39_001_091614.bin", "last mod"=timestamp(3493762659 s since 1904-01-01), "file name str"="D:\\Data\\Ultrasound\\LSCO\\LSCO22__130814c\\5_Cooling_2nd_try\\September_2014\\091614\\103.18900K_500_2500_2.10000V_0.00000T_Sep16-2014__21-37-39_001_091614.bin", "mod time(min)"=58229377.65, "file format"=enum."binary", "power(V)"=2.1, "Magn Field(T) "=0.0}, {"temperature"=103.003, "temperature str"="103.00300", "file path"=path "D:/Data/Ultrasound/LSCO/LSCO22__130814c/5_Cooling_2nd_try/September_2014/091614/103.00300K_500_2500_2.10000V_0.00000T_Sep16-2014__21-38-58_001_091614.bin", "last mod"=timestamp(3493762738 s since 1904-01-01), "file name str"="D:\\Data\\Ultrasound\\LSCO\\LSCO22__130814c\\5_Cooling_2nd_try\\September_2014\\091614\\103.00300K_500_2500_2.10000V_0.00000T_Sep16-2014__21-38-58_001_091614.bin", "mod time(min)"=58229378.96666667, "file format"=enum."binary", "power(V)"=2.1, "Magn Field(T) "=0.0}, {"temperature"=102.827, "temperature str"="102.82700", "file path"=path "D:/Data/Ultrasound/LSCO/LSCO22__130814c/5_Cooling_2nd_try/September_2014/091614/102.82700K_500_2500_2.10000V_0.00000T_Sep16-2014__21-40-17_001_091614.bin", "last mod"=timestamp(3493762817 s since 1904-01-01), "file name str"="D:\\Data\\Ultrasound\\LSCO\\LSCO22__130814c\\5_Cooling_2nd_try\\September_2014\\091614\\102.82700K_500_2500_2.10000V_0.00000T_Sep16-2014__21-40-17_001_091614.bin", "mod time(min)"=58229380.28333333, "file format"=enum."binary", "power(V)"=2.1, "Magn Field(T) "=0.0}, {"temperature"=102.644, "temperature str"="102.64400", "file path"=path "D:/Data/Ultrasound/LSCO/LSCO22__130814c/
